vi "Comp_32_Elements.vi"(10 "Array":u16[](array[numeric])=[0, 0, 0, 0, 0, 0, 0, 0, 0, 0, 0, 0, 0, 0, 0, 0, 0, 0, 0, 0, 0, 0, 0, 0, 0, 0, 0, 0, 0, 0, 0, 0], 11 "CompVal":u16) -> (3 "Result":bool)   [LabVIEW 2016]
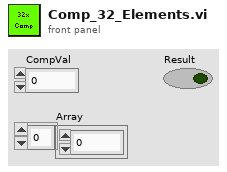
[diagram p1: front panel]
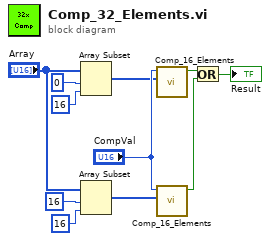
[diagram p0: block diagram]
diagram:
  n1 = Array Subset(array="Array", index=0, length=16) -> (w3:u16[])
  n2 = Array Subset(array="Array", index=16, length=16) -> (w7:u16[])
  n3 = call "Comp_16_Elements.vi"("Array"=w3, "CompVal"="CompVal") -> ("result"=w9:bool)  [unwired: 9 in]
  n4 = call "Comp_16_Elements.vi"("Array"=w7, "CompVal"="CompVal") -> ("result"=w10:bool)  [unwired: 9 in]
  n5 = Or(x=w9, y=w10) -> (x .or. y?=→"Result":bool)
